vi "Save VI at Path.vi"(5 "Save a Copy (F)":bool, 6 "Without Diagram (F)":bool, 7 "Override Existing? (T)":bool=TRUE, 8 "error in (no error)":errorcluster, 10 "Path":path, 11 "VI in":refnum<vi>) -> (0 "error out":errorcluster, 3 "VI out":refnum<vi>)   [LabVIEW 2019, in "VI Scripting Tools.lvlib"]
uses:
  VI Scripting Tools.lvlib
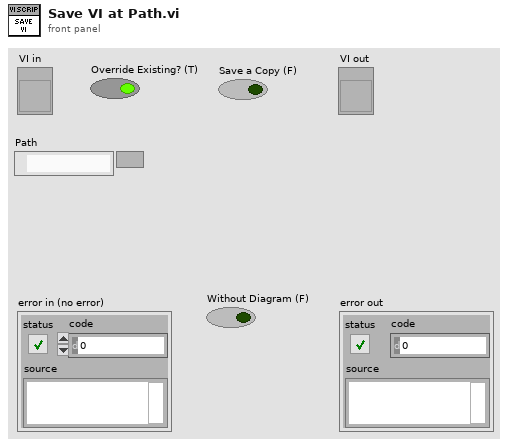
[diagram p1: front panel]
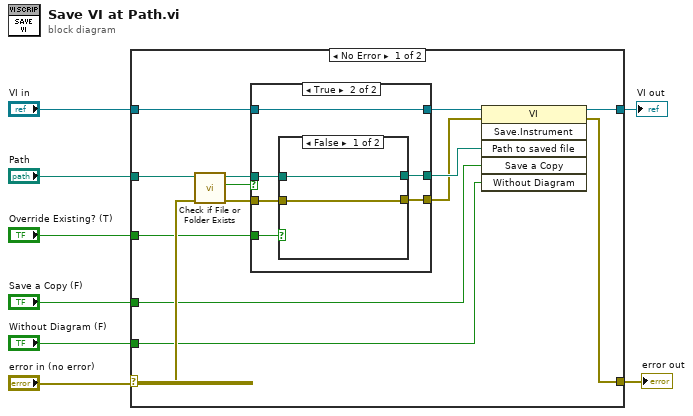
[diagram p0: block diagram]
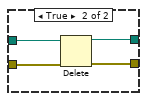
[diagram p3: hidden frame]
diagram:
  n1 = case shown="No Error" "error in (no error)" {
    selector: "error in (no error)" -> [w20 w38]
    tunnel: "Path" -> [w21 _]
    tunnel: "VI in" -> [w22 w39]
    tunnel: [w9 w38] -> w6
    tunnel: [w15 w39] -> w5
    tunnel: "Save a Copy (F)" -> [w11 _]
    tunnel: "Without Diagram (F)" -> [w10 _]
    tunnel: "Override Existing? (T)" -> [w13 _]
    frame No Error {
      n2 = call <vilib>:"Check if File or Folder Exists.vi"("error in (no error)"=w20, "path"=w21) -> ("error out"=w17:errorcluster, "file or folder exists?"=w18:bool, "dup path"=w19:path)  [unwired: 7 in]
      n3 = case shown="True" w18 {
        tunnel: w22 -> [w25 w31]
        tunnel: [w25 w31] -> w16
        tunnel: w19 -> [w23 w30]
        tunnel: w17 -> [w24 w29]
        tunnel: [w23 w28] -> w14
        tunnel: [w24 w27] -> w12
        tunnel: w13 -> [_ w26]
        frame False {
        }
        frame True {
          n4 = case shown="False" w26 {
            tunnel: w30 -> [w33 w37]
            tunnel: w29 -> [w32 w36]
            tunnel: [w33 w35] -> w28
            tunnel: [w32 w34] -> w27
            frame False {
            }
            frame True {
              n5 = Delete(path (use dialog)=w37, error in=w36) -> (deleted path=w35:path, error out=w34:errorcluster)  [unwired: 3 in, 1 out]
            }
          }
        }
      }
      n6 = invoke class="VI" method="Save.Instrument"(reference=w16, error in=w12, "Path to saved file"=w14, "Save a Copy"=w11, "Without Diagram"=w10) -> (reference out=w15:refnum<vi>, error out=w9:errorcluster)  [unwired: 1 in, 4 out]
    }
    frame Error {
    }
  }
  "error out" <- w6
  "VI out" <- w5
